vi "CalcRobotRectangle.vi"(10 "Position":cluster{"X":dbl, "Y":dbl, "Angle":dbl}) -> (2 "line endpoints":cluster{"x":i16, "y":i16}[](array[cluster])=[{"x"=50, "y"=75}, {"x"=50, "y"=135}, {"x"=100, "y"=135}, {"x"=120, "y"=75}])   [LabVIEW 2009, in "Host.lvlib" / "Draw.lvlib"]
uses:
  Draw.lvlib
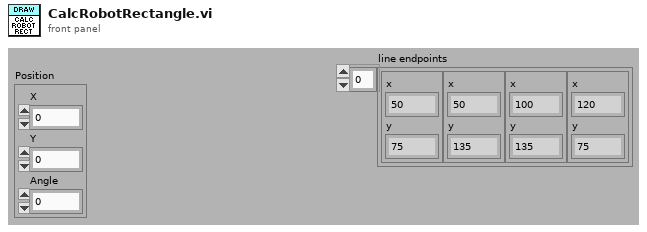
[diagram p1: front panel]
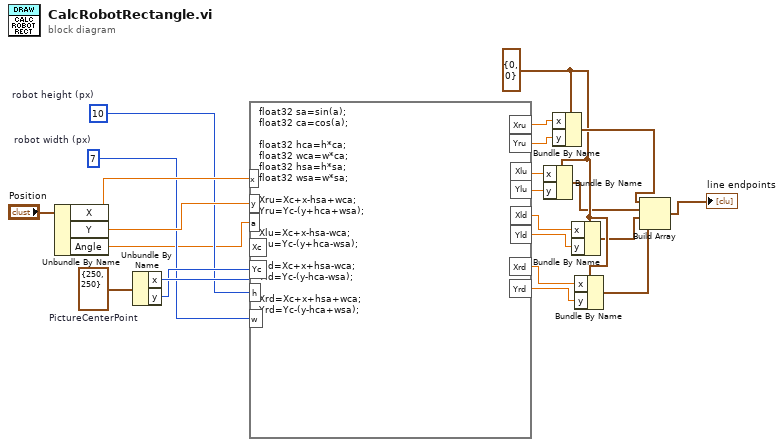
[diagram p0: block diagram]
diagram:
  w6 = cluster{"x":i32, "y":i32} {"x"=0, "y"=0}
  w23 = cluster{"x":i32, "y":i32} {"x"=250, "y"=250}  # PictureCenterPoint
  w16 = 7  # robot width (px)
  w17 = 10  # robot height (px)
  n1 = Unbundle By Name("Position") -> ("X"=w21:dbl, "Y"=w20:dbl, "Angle"=w15:dbl)
  n2 = Unbundle By Name(w23) -> ("x"=w19:i32, "y"=w18:i32)
  n3 = formula code="float32 sa=sin(a);\nfloat32 ca=cos(a);\n\nfloat32 hca=h*ca;\nfloat32 wca=w*ca;\nfloat32 hsa=h*sa;\nfloat32 wsa=w*sa;\n\nXru=Xc+x-hsa+wca;\nYru=Yc-(y+hca+wsa);\n\nXlu=Xc+x-hsa-wca;\nYlu=Yc-(y+hca-wsa);\n\nXld=Xc+x+hsa-wca;\nYld=Yc-(y-hca-wsa);\n\nXrd=Xc+x+hsa+wca;\nYrd=Yc-(y-hca+wsa);"("x"=w21, "y"=w20, "Xc"=w19, "Yc"=w18, "h"=w17, "w"=w16, "a"=w15) -> ("Xru"=w14:dbl, "Yru"=w13:dbl, "Xlu"=w10:dbl, "Xld"=w8:dbl, "Xrd"=w5:dbl, "Ylu"=w9:dbl, "Yld"=w7:dbl, "Yrd"=w4:dbl)
  n4 = Bundle By Name(cluster=w6, "x"=w10, "y"=w9) -> (w3:cluster{"x":i32, "y":i32})
  n5 = Bundle By Name(cluster=w6, "x"=w14, "y"=w13) -> (w12:cluster{"x":i32, "y":i32})
  n6 = Bundle By Name(cluster=w6, "x"=w8, "y"=w7) -> (w2:cluster{"x":i32, "y":i32})
  n7 = Bundle By Name(cluster=w6, "x"=w5, "y"=w4) -> (w1:cluster{"x":i32, "y":i32})
  n8 = Build Array(w12, w3, w2, w1) -> (→"line endpoints":cluster{"x":i32, "y":i32}[])
